vi "Timeseries to Array.vi"(11 "Waveform New":cluster{dbl, dbl, dbl[][]}) -> (3 "?":dbl[][](array[numeric]))   [LabVIEW 2017]
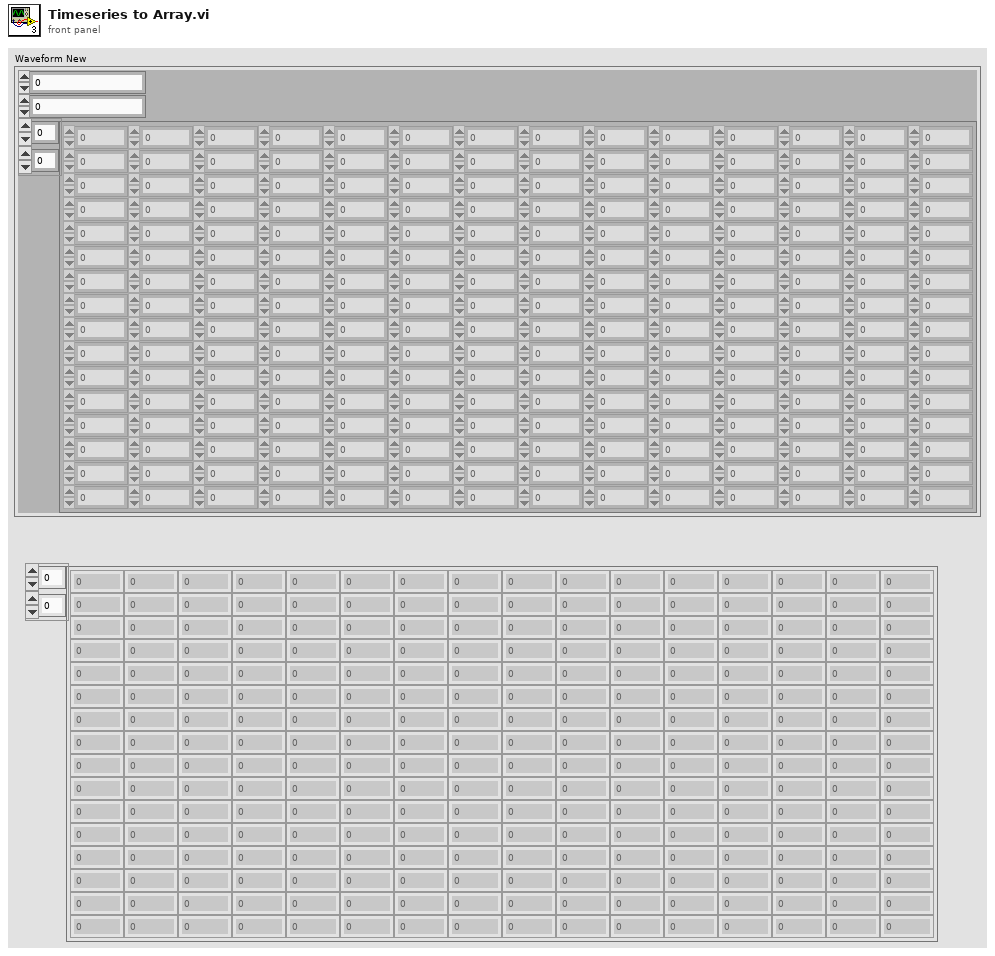
[diagram p1: front panel]
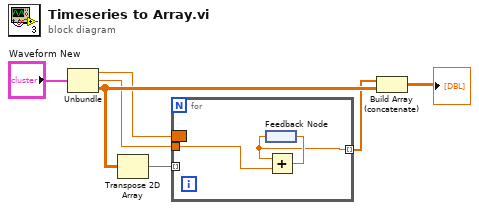
[diagram p0: block diagram]
diagram:
  n1 = Unbundle("Waveform New") -> (w4:dbl, w5:dbl, w6:dbl[][])
  n2 = Transpose 2D Array(2D array=w6) -> (transposed array=w1:dbl[][])
  n3 = for {
    tunnel: w1 -> [_] mode=indexing
    tunnel: w5 -> [w10]
    border: w4 -> [_]
    tunnel: [w8] -> w3 mode=indexing
    n4 = feedback #1() -> (w8:dbl)
    n5 = Add(x=w8, y=w10) -> (x+y=w9:dbl)
    n6 = feedback-in #1(w9) -> ()
  }
  n7 = Build Array (concatenate)(w3, w6) -> (→"?":dbl[][])
